vi "Telescope Read Current Status.vi"(8 "error in (no error)":errorcluster, 11 "Telescope Simulator in":refnum<class "Telescope Simulator.lvclass">) -> (0 "error out":errorcluster, 1 "Raw Response":string, 2 "Telescope Status":T1, 3 "Telescope Simulator out":refnum<class "Telescope Simulator.lvclass">, 4 "Cmd Sent":string)   [LabVIEW 2024, in "Telescope Simulator.lvclass"]
uses:
  Telescope Simulator.lvclass
  Telescope cluster Status.ctl
  typedefs/CC cluster RA and DEC.ctl
  Telescope enum Status.ctl
  Telescope Simulator.lvclass/Telescope Simulator.ctl
  Telescope.lvclass
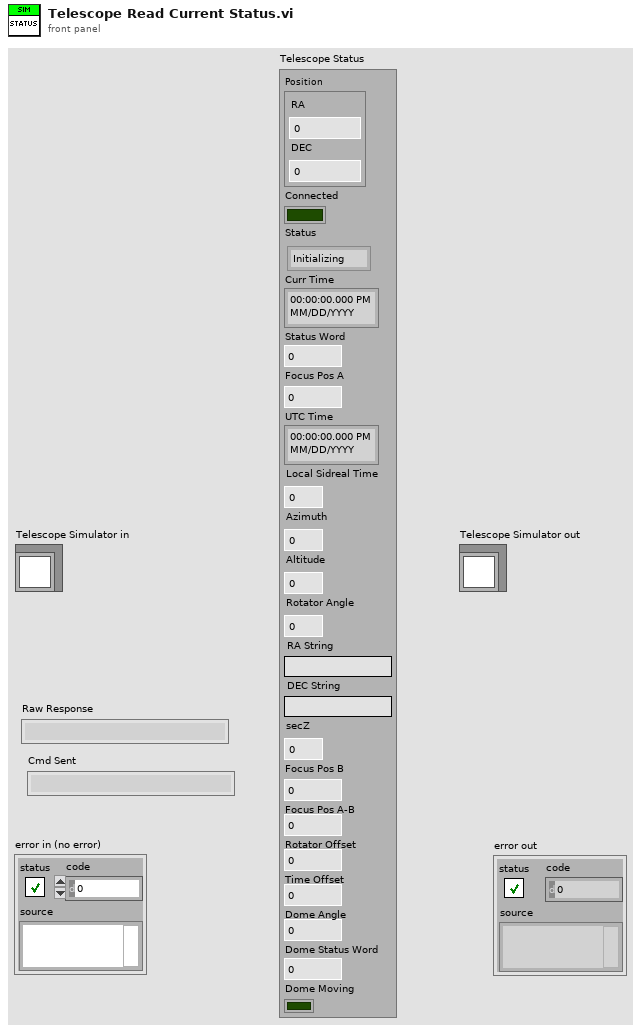
[diagram p1: front panel]
types:
  T1 = typedef "Telescope.lvclass/Telescope cluster Status.ctl" = cluster{"Position":T2, "Connected":bool, "Status":T3, "Curr Time":timestamp, "Status Word":u32, "Focus Pos A":dbl, "UTC Time":timestamp, "Local Sidreal Time":dbl, "Azimuth":dbl, "Altitude":dbl, "Rotator Angle":dbl, "RA String":string, "DEC String":string, "secZ":dbl, "Focus Pos B":dbl, "Focus Pos A-B":dbl, "Rotator Offset":dbl, "Time Offset":dbl, "Dome Angle":dbl, "Dome Status Word":u32, "Dome Moving":bool}
  T2 = typedef "CC cluster RA and DEC.ctl" = cluster{"RA":dbl, "DEC":dbl}
  T3 = typedef "Telescope.lvclass/Telescope enum Status.ctl" = enum16{"Initializing", "Ready", "Moving", "Focusing", "Error"}
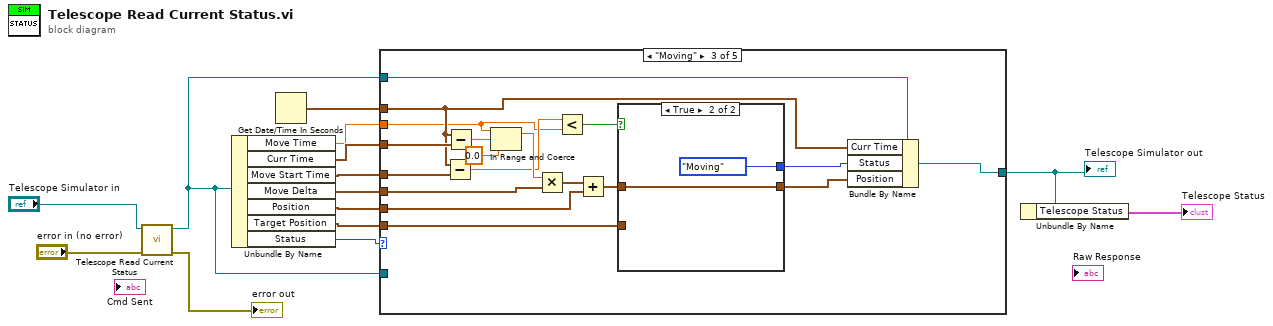
[diagram p0: block diagram]
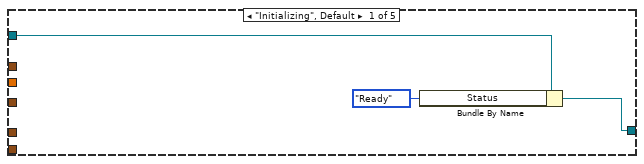
[diagram p2: hidden frame]
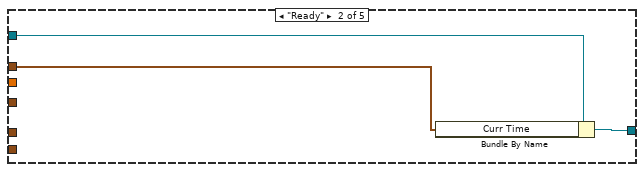
[diagram p3: hidden frame]
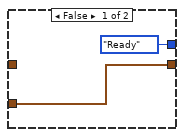
[diagram p4: hidden frame]
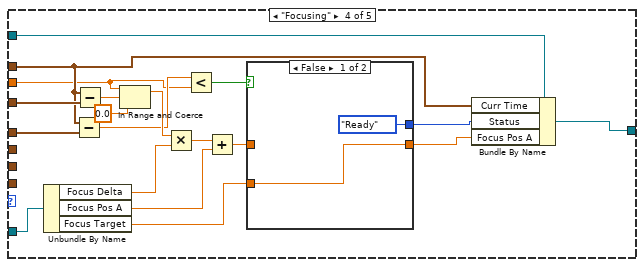
[diagram p5: hidden frame]
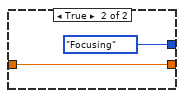
[diagram p6: hidden frame]
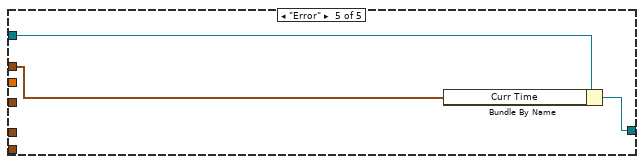
[diagram p7: hidden frame]
diagram:
  n1 = call-parent "Telescope Read Current Status.vi"("error in (no error)"="error in (no error)", "Telescope in"="Telescope Simulator in") -> ("error out"=→"error out":errorcluster, "Telescope out"=w1:refnum<class "Telescope Simulator.lvclass">)  [unwired: 5 in, 3 out]
  n2 = Unbundle By Name(w1) -> ("Move Time"=w2:dbl, "Curr Time"=w3:timestamp, "Move Start Time"=w10:timestamp, "Move Delta"=w9:T2, "Position"=w8:T2, "Target Position"=w7:T2, "Status"=w4:T3)
  n3 = Get Date/Time In Seconds() -> (seconds since 1Jan1904=w11:timestamp)
  n4 = case shown="\"Moving\"" w4 {
    tunnel: w11 -> [_ w19 w25 w51 w67]
    tunnel: w10 -> [_ _ w24 w50 _]
    tunnel: w1 -> [w17 w20 w38 w61 w68]
    tunnel: w9 -> [_ _ w37 _ _]
    tunnel: w8 -> [_ _ w35 _ _]
    tunnel: w7 -> [_ _ w28 _ _]
    tunnel: [w15 w18 w27 w53 w66] -> w5
    tunnel: w3 -> [_ _ w26 w52 _]
    tunnel: w2 -> [_ _ w21 w47 _]
    tunnel: w1 -> [_ _ _ w46 _]
    frame "Initializing", Default {
      n5 = Bundle By Name(cluster=w17, "Status"=Telescope_enum_Status."Ready" ("Telescope Status.Status")) -> (w15:refnum<class "Telescope Simulator.lvclass">)
    }
    frame "Ready" {
      n6 = Bundle By Name(cluster=w20, "Curr Time"=w19) -> (w18:refnum<class "Telescope Simulator.lvclass">)
    }
    frame "Moving" {
      n7 = Subtract(x=w25, y=w24) -> (x-y=w23:dbl)
      n8 = Subtract(x=w25, y=w26) -> (x-y=w34:dbl)
      n9 = In Range and Coerce(upper limit=w21, x=w34, lower limit=0.0) -> (coerced(x)=w32:dbl)  [unwired: 1 out]
      n10 = Multiply(x=w32, y=w37) -> (x*y=w36:T2)
      n11 = Less?(x=w23, y=w21) -> (x < y?=w22:bool)
      n12 = Add(x=w36, y=w35) -> (x+y=w31:T2)
      n13 = case shown="True" w22 {
        tunnel: w31 -> [_ w42]
        tunnel: [w40 w42] -> w30
        tunnel: [Telescope_enum_Status."Ready" ("Telescope Status.Status") Telescope_enum_Status."Moving" ("Telescope Status.Status")] -> w29
        tunnel: w28 -> [w40 _]
        frame False {
        }
        frame True {
        }
      }
      n14 = Bundle By Name(cluster=w38, "Curr Time"=w25, "Status"=w29, "Position"=w30) -> (w27:refnum<class "Telescope Simulator.lvclass">)
    }
    frame "Focusing" {
      n15 = Unbundle By Name(w46) -> ("Focus Delta"=w45:dbl, "Focus Pos A"=w44:dbl, "Focus Target"=w43:dbl)
      n16 = Subtract(x=w51, y=w50) -> (x-y=w49:dbl)
      n17 = Subtract(x=w51, y=w52) -> (x-y=w59:dbl)
      n18 = In Range and Coerce(upper limit=w47, x=w59, lower limit=0.0) -> (coerced(x)=w57:dbl)  [unwired: 1 out]
      n19 = Multiply(x=w57, y=w45) -> (x*y=w60:dbl)
      n20 = Less?(x=w49, y=w47) -> (x < y?=w48:bool)
      n21 = Add(x=w60, y=w44) -> (x+y=w56:dbl)
      n22 = case shown="False" w48 {
        tunnel: w56 -> [_ w65]
        tunnel: [w63 w65] -> w55
        tunnel: [Telescope_enum_Status."Ready" ("Telescope Status.Status") Telescope_enum_Status."Focusing" ("Telescope Status.Status")] -> w54
        tunnel: w43 -> [w63 _]
        frame False {
        }
        frame True {
        }
      }
      n23 = Bundle By Name(cluster=w61, "Curr Time"=w51, "Status"=w54, "Focus Pos A"=w55) -> (w53:refnum<class "Telescope Simulator.lvclass">)
    }
    frame "Error" {
      n24 = Bundle By Name(cluster=w68, "Curr Time"=w67) -> (w66:refnum<class "Telescope Simulator.lvclass">)
    }
  }
  "Telescope Simulator out" <- w5
  n25 = Unbundle By Name(w5) -> ("Telescope Status"=→"Telescope Status":T1)
